vi "solar Msg Voyager (HS).vi"(8 "error in (no error)":errorcluster, 11 "solar in":refnum<class "solar.lvclass">) -> (0 "error out":errorcluster, 3 "solar out":refnum<class "solar.lvclass">)   [LabVIEW 2018]
doc: "This handles the Voyager 'HANDSHAKE' back to COSMOS. The LINC interface requires the HDR_GUID as part of the telemetry returned. If an error exists, this also returns the 'ERROR' packet."
uses:
  solar.lvclass
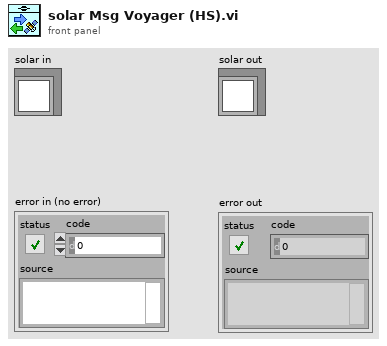
[diagram p1: front panel]
types:
  T1 = typedef "solar_voy_ctl Voyager Refnum.ctl" = refnum<k1>
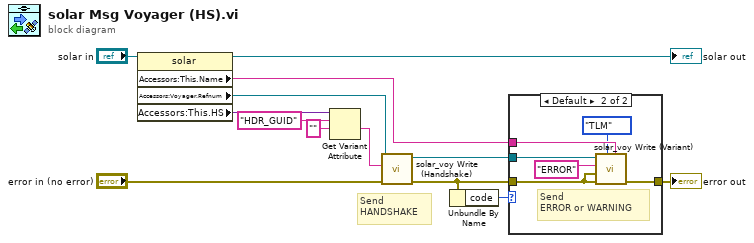
[diagram p0: block diagram]
diagram:
  # "Send\nHANDSHAKE"
  n1 = property class="solar"(reference="solar in") -> (reference out=→"solar out":refnum<class "solar.lvclass">, "Accessors:This.Name"=w4:string, "Accessors:Voyager.Refnum"=w10:T1, "Accessors:This.HS"=w9:variant)  [unwired: 1 in, 1 out]
  n2 = Get Variant Attribute(Variant=w9, name="HDR_GUID", default value (empty Variant)="") -> (value=w6:string)  [unwired: 1 in, 3 out]
  n3 = call "solar_voy Write (Handshake).vi"("error in (no error)"="error in (no error)", "HDR_GUID"=w6, "Voyager Refnum in"=w10) -> ("error out"=w2:errorcluster, "Voyager Refnum out"=w5:T1)  [unwired: 7 in]
  n4 = Unbundle By Name(w2) -> ("code"=w1:i32)
  n5 = case shown="Default" w1 {
    tunnel: w5 -> [_ w20]
    tunnel: w4 -> [_ w19]
    tunnel: w2 -> [w14 w18]
    tunnel: [w14 w17] -> w3
    frame 0 {
    }
    frame Default {
      # "Send\nERROR or WARNING"
      n6 = call "solar_voy Write (Variant).vi"("TARGET"=w19, "CMD"=enum8{"CMD", "TLM"}."TLM", "error in (no error)"=w18, "Variant (No HDR)"=w18, "PACKET (\"\" = Use Variant)"="ERROR" ("PACKET (\"\" = Use Variant)"), "Voyager Refnum in"=w20) -> ("error out"=w17:errorcluster)  [unwired: 4 in, 1 out]
    }
  }
  "error out" <- w3
